vi "Load Model.vi"(0 "reference in":refnum<class "Battery.lvclass">, 2 "Model Parameters":T1={"chemistry"="Chen2020", "model_type"="SPMe"}, 5 "Error In":errorcluster) -> (14 "reference out":refnum<class "Battery.lvclass">, 16 "model loaded":bool, 19 "Error Out":errorcluster)   [LabVIEW 2023, in "Battery.lvclass"]
uses:
  Battery.lvclass
  Model Parameters.ctl
  Battery.lvclass/Battery.ctl
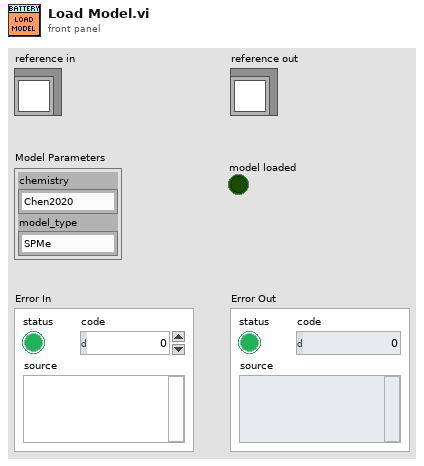
[diagram p1: front panel]
types:
  T1 = typedef "Battery.lvclass/Model Parameters.ctl" = cluster{"chemistry":string, "model_type":string}
  T2 = typedef "Battery.lvclass/ObjectAttributes.ctl" = cluster{"Python module":path, "Python Session":refnum<k35>, "PybammWrapper":refnum<k38>, "model loaded":bool, "simulation loaded":bool, "simulation enabled":bool, "SOC OCV Curve":dbl[][], "Open Circuit Voltage (V)":dbl, "State of Charge (%)":dbl, "HPS17K Refs":refnum<class "HPS-17000.lvclass">[], "# Cells in Series":u16, "# Cells in Parallel":u16, "Model Parameters":T1, "Simulation Parameters":T3}
  T3 = typedef "Battery.lvclass/Simulation Parameters.ctl" = cluster{"num_rc_pairs":i32, "R0":dbl, "R1":dbl, "C1":dbl, "R2":dbl, "C2":dbl, " nominal_capacity_Ah":dbl, "upper_voltage_cutoff":dbl, "lower_voltage_cutoff":dbl}
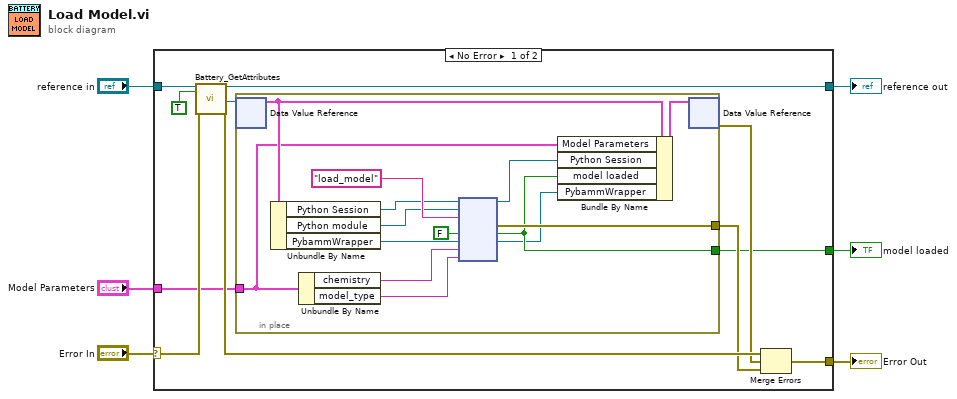
[diagram p0: block diagram]
diagram:
  n1 = case shown="No Error" "Error In" {
    selector: "Error In" -> [w16 w33]
    tunnel: [w14 w33] -> w5
    tunnel: [w15 w32] -> w3
    tunnel: "reference in" -> [w17 w32]
    tunnel: "Model Parameters" -> [w9 _]
    tunnel: [w7 _] -> w1
    frame No Error {
      n2 = call "Battery_GetAttributes.vi"("reference in"=w17, "OnlyGetDvrReference(False)"=TRUE, "Error In"=w16) -> ("reference out"=w15:refnum<class "Battery.lvclass">, "DataRef"=w13:refnum<data-value>, "Error Out"=w11:errorcluster)  [unwired: 13 in, 1 out]
      n3 = in-place {
        in-place-border: w9 -> [w18]
        in-place-border: [w22] -> w8
        in-place-border: [w21] -> w7
        n4 = in-place-dvr #1(w13) -> (w30:T2)  [unwired: 1 out]
        n5 = Unbundle By Name(w30) -> ("Python Session"=w24:refnum<k35>, "Python module"=w23:path, "PybammWrapper"=w25:refnum<k38>)
        n6 = Unbundle By Name(w18) -> ("chemistry"=w28:string, "model_type"=w29:string)
        n7 = node(w24, w23, "load_model" ("function name"), FALSE, w25, w28, w29) -> (w19:refnum<k35>, w22:errorcluster, w21:bool, w20:refnum<k38>)  [unwired: 3 in, 2 out]
        n8 = Bundle By Name(cluster=w30, "Model Parameters"=w18, "Python Session"=w19, "model loaded"=w21, "PybammWrapper"=w20) -> (w31:T2)
        n9 = in-place-dvr #1(w31) -> (w10:errorcluster)  [unwired: 1 out]
      }
      n10 = Merge Errors(w11, w10, w8) -> (w14:errorcluster)
    }
    frame Error {
    }
  }
  "Error Out" <- w5
  "reference out" <- w3
  "model loaded" <- w1
